vi "Agilent VNA Set Cal Off.vi"(6 "Channel":i8=1 min=1 max=99 step=1, 7 "Agilent VNA":T1, 8 "error in (no error)":errorcluster, 11 "VISA Resource Name":refnum<visa-resource-name>) -> (0 "error out":errorcluster {"code" format="%.0x"}, 3 "dup VISA Resource Name":refnum<visa-resource-name>)   [LabVIEW 2011]
doc: "This Vi for the HP8753B Network Analyzer is used to set averaging, smoothing, and the IF bandwidth."
uses:
  TypeDefs/Agilent VNA Instrument Info.ctl
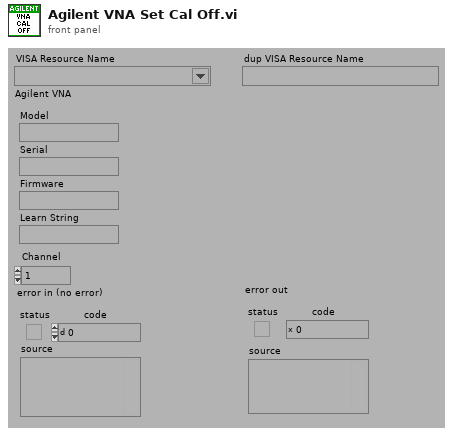
[diagram p1: front panel]
types:
  T1 = typedef "Agilent VNA Instrument Info.ctl" = cluster{"Model":string, "Serial":string, "Firmware":string, "Learn String":string}
  T2 = typedef "Agilent VNA Model.ctl" = enum16{"Not Supported", "8510X", "8719X", "8720X", "8722X", "8753X", "ENA", "PNA", "Field Fox"}
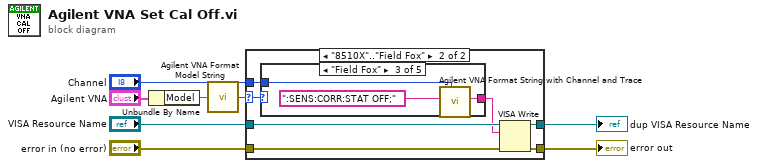
[diagram p0: block diagram]
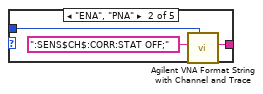
[diagram p4: hidden frame]
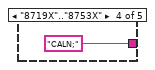
[diagram p5: hidden frame]
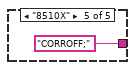
[diagram p6: hidden frame]
diagram:
  n1 = Unbundle By Name("Agilent VNA") -> ("Model"=w3:string)
  n2 = call "Agilent VNA Format Model String.vi"("Model"=w3) -> ("Model"=w2:T2)
  n3 = case shown="\"8510X\"..\"Field Fox\"" w2 {
    selector: w2 -> [_ w11]
    tunnel: "VISA Resource Name" -> [w10 w17]
    tunnel: "error in (no error)" -> [w9 w16]
    tunnel: [w9 w15] -> w6
    tunnel: "Channel" -> [_ w12]
    tunnel: [w10 w14] -> w1
    frame "Not Supported" {
    }
    frame "8510X".."Field Fox" {
      n4 = case shown="\"Field Fox\"" w11 {
        tunnel: [_ w19 w22 "CALN;" "CORROFF;"] -> w13
        tunnel: w12 -> [_ w18 w21 _ _]
        frame "Not Supported" {
        }
        frame "ENA", "PNA" {
          n5 = call "Agilent VNA Format String with Channel and Trace.vi"("Channel"=w18, "String"=":SENS$CH$:CORR:STAT OFF;") -> ("String Out"=w19:string)  [unwired: 1 in, 6 out]
        }
        frame "Field Fox" {
          n6 = call "Agilent VNA Format String with Channel and Trace.vi"("Channel"=w21, "String"=":SENS:CORR:STAT OFF;") -> ("String Out"=w22:string)  [unwired: 1 in, 6 out]
        }
        frame "8719X".."8753X" {
        }
        frame "8510X" {
        }
      }
      n7 = VISA Write(VISA resource name=w17, write buffer=w13, error in (no error)=w16) -> (VISA resource name out=w14:refnum<visa-resource-name>, error out=w15:errorcluster)  [unwired: 1 out]
    }
  }
  "error out" <- w6
  "dup VISA Resource Name" <- w1
